vi "Account FGV.vi"(7 "账户方法":T1, 8 "错误输入":cluster{"状态":bool, "代码":i32, "源":string}, 11 "量":dbl) -> (0 "错误输出":cluster{"状态":bool, "代码":i32, "源":string}, 3 "账户余额":dbl)   [LabVIEW 2012]
uses:
  Account Methods.ctl
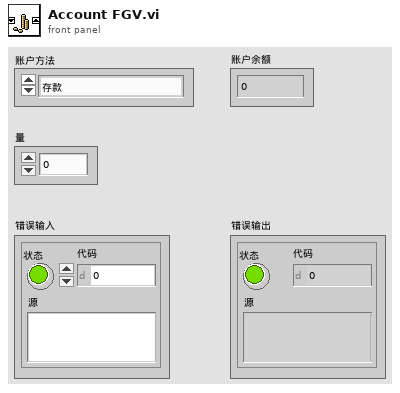
[diagram p1: front panel]
types:
  T1 = typedef "Account Methods.ctl" = enum16{"存款", "取款", "查询余额", "结清余额"}
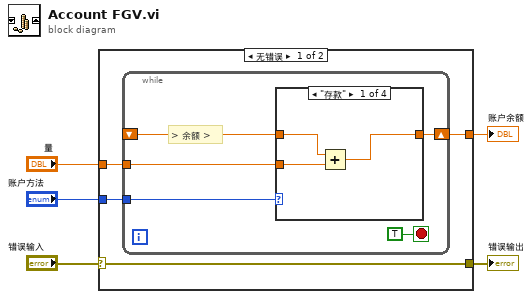
[diagram p0: block diagram]
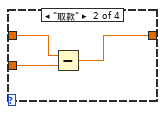
[diagram p2: hidden frame]
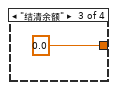
[diagram p3: hidden frame]
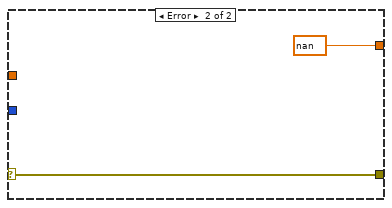
[diagram p5: hidden frame]
diagram:
  n1 = case shown="无错误" "错误输入" {
    selector: "错误输入" -> [w6 w24]
    tunnel: "量" -> [w9 _]
    tunnel: "账户方法" -> [w8 _]
    tunnel: [w7 sgl nan] -> w3
    tunnel: [w6 w24] -> w1
    frame No Error {
      n2 = while {
        shift-right: [w12] -> w7
        shift-left: _ -> [w13]
        tunnel: w9 -> [w11]
        tunnel: w8 -> [w10]
        stop <- TRUE stop-if-true
        # "> 余额 >"
        n3 = case shown="\"存款\"" w10 {
          tunnel: w11 -> [w17 w20 _ _]
          tunnel: w13 -> [w16 w19 _ w22]
          tunnel: [w15 w18 0.0 w22] -> w12
          frame "存款" {
            n4 = Add ("加")(x=w16, y=w17) -> (x+y=w15:dbl)
          }
          frame "取款" {
            n5 = Subtract ("减")(x=w19, y=w20) -> (x-y=w18:dbl)
          }
          frame "结清余额" {
          }
          frame "查询余额" {
          }
        }
      }
    }
    frame Error {
    }
  }
  "错误输出" <- w1
  "账户余额" <- w3
